vi "Get_Array_Subset.vi"(5 "String Array In":string[](array[string]), 6 "Subset Name":string) -> (0 "index after match":i32, 1 "Array Subset Out":string[](array[string]), 2 "Empty Subset?":bool, 3 "Length before match":i32, 4 "First Element":string)   [LabVIEW 2010]
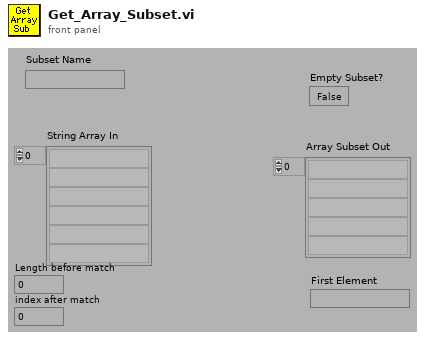
[diagram p1: front panel]
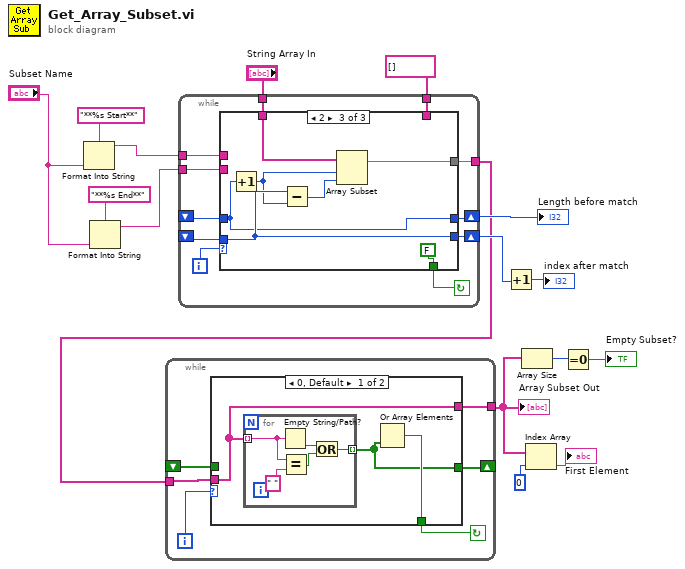
[diagram p0: block diagram]
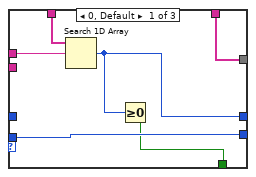
[diagram p2: hidden frame]
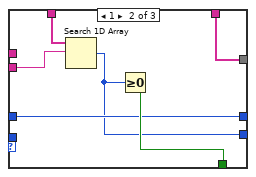
[diagram p3: hidden frame]
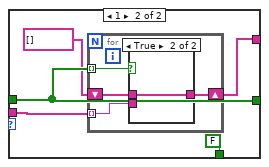
[diagram p4: hidden frame]
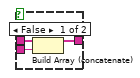
[diagram p5: hidden frame]
diagram:
  n1 = Format Into String(format string="**%s Start**" ("Format String"), "Subset Name") -> (resulting string=w12:string)  [unwired: 2 in, 1 out]
  n2 = Format Into String(format string="**%s End**" ("Format String"), "Subset Name") -> (resulting string=w10:string)  [unwired: 2 in, 1 out]
  n3 = while {
    tunnel: w10 -> [w18]
    shift-left: _ -> [w20]
    shift-right: [w19] -> w6
    shift-left: _ -> [w17]
    shift-right: [w21] -> w7
    tunnel: string[] [] ("Array Subset Out") -> [w22]
    tunnel: [w23] -> w4
    tunnel: w12 -> [w26]
    tunnel: "String Array In" -> [w27]
    i -> [w25]
    stop <- w24 continue-if-true
    n4 = case shown="2" w25 {
      tunnel: w27 -> [w33 w39 w42]
      tunnel: w26 -> [w32 _ _]
      tunnel: [w28 w37 FALSE] -> w24
      tunnel: [w31 w38 w43] -> w23
      tunnel: w22 -> [w31 w38 _]
      tunnel: [w29 w35 w41] -> w21
      tunnel: w20 -> [w30 _ w45]
      tunnel: [w30 w34 w45] -> w19
      tunnel: w18 -> [_ w36 _]
      tunnel: w17 -> [_ w35 w41]
      frame 0, Default {
        n5 = Search 1D Array(1D array=w33, element=w32) -> (index of element=w29:i32)  [unwired: 1 out]
        n6 = Greater Or Equal To 0?(x=w29) -> (x >= 0?=w28:bool)
      }
      frame 1 {
        n7 = Search 1D Array(1D array=w39, element=w36) -> (index of element=w34:i32)  [unwired: 1 out]
        n8 = Greater Or Equal To 0?(x=w34) -> (x >= 0?=w37:bool)
      }
      frame 2 {
        n9 = Increment(x=w41) -> (x+1=w40:i32)
        n10 = Subtract(x=w45, y=w40) -> (x-y=w46:i32)
        n11 = Array Subset(array=w42, index=w40, length=w46) -> (w43:string[])
      }
    }
  }
  "Length before match" <- w7
  n12 = while {
    shift-left: _ -> [w47]
    shift-right: [w48] -> _
    tunnel: [w49] -> w2
    tunnel: w4 -> [w51]
    i -> [w52]
    stop <- w50 continue-if-true
    n13 = case shown="0, Default" w52 {
      tunnel: w51 -> [w54 w62]
      tunnel: [w55 FALSE] -> w50
      tunnel: [w54 w65] -> w49
      tunnel: [w53 w64] -> w48
      tunnel: w47 -> [_ w64]
      frame 0, Default {
        n14 = for {
          tunnel: w54 -> [w59] mode=indexing
          tunnel: [w56] -> w53 mode=indexing
          n15 = Empty String/Path?(string/path=w59) -> (empty?=w57:bool)
          n16 = Equal?(x=w59, y=" ") -> (x = y?=w58:bool)
          n17 = Or(x=w57, y=w58) -> (x .or. y?=w56:bool)
        }
        n18 = Or Array Elements(Boolean array=w53) -> (logical OR=w55:bool)
      }
      frame 1 {
        n19 = for {
          shift-right: [w68] -> w65
          shift-left: string[] [] -> [w67]
          tunnel: w64 -> [w69] mode=indexing
          tunnel: w62 -> [w66] mode=indexing
          n20 = case shown="True" w69 {
            tunnel: [w71 w73] -> w68
            tunnel: w67 -> [w72 w73]
            tunnel: w66 -> [w70 _]
            frame False {
              n21 = Build Array (concatenate)(w72, w70) -> (w71:string[])
            }
            frame True {
            }
          }
        }
      }
    }
  }
  "Array Subset Out" <- w2
  n22 = Increment(x=w6) -> (x+1=→"index after match":i32)
  n23 = Array Size(array=w2) -> (size(s)=w9:i32)
  n24 = Index Array(array=w2, index=0 ("Index")) -> (element=→"First Element":string)
  n25 = Equal To 0?(x=w9) -> (x = 0?=→"Empty Subset?":bool)
